vi "VectorField1008.vi"   [LabVIEW 2013]
uses:
  <vilib>/Heliosphere Research LLC/Advanced Plotting Toolkit/api_plotting/VectorFieldProperties.ctl
  <vilib>/Heliosphere Research LLC/Advanced Plotting Toolkit/typedefs/PlotColor.ctl
  <vilib>/Heliosphere Research LLC/Advanced Plotting Toolkit/properties/Colormap.ctl
  <vilib>/Heliosphere Research LLC/Advanced Plotting Toolkit/properties/Colormap_Map.ctl
  <vilib>/Heliosphere Research LLC/Advanced Plotting Toolkit/properties/Colormap_Scaling.ctl
  <vilib>/Heliosphere Research LLC/Advanced Plotting Toolkit/properties/Display.ctl
  <vilib>/Heliosphere Research LLC/Advanced Plotting Toolkit/Advanced Plotting Toolkit.lvlib
types:
  T1 = typedef "Advanced Plotting Toolkit.lvlib/Colormap_Map.ctl" = enum16{"Automatic", "Rainbow", "Hot and Cold", "White-Black", "White-Blue", "White-Green", "White-Red", "Fire", "Water", "Earth", "Air", "Pastel", "Banded", "Stepped"}
  T2 = typedef "Advanced Plotting Toolkit.lvlib/VectorFieldProperties.ctl" = cluster{"Color":T3, "Arrow Scale":dbl, "Colormap":T4, "Display":T6}
  T3 = typedef "Advanced Plotting Toolkit.lvlib/PlotColor.ctl" = u32
  T4 = typedef "Advanced Plotting Toolkit.lvlib/Colormap.ctl" = cluster{"Map":T1, "Value Min":dbl, "Value Max":dbl, "Scaling":T5, "Reverse":bool}
  T5 = typedef "Advanced Plotting Toolkit.lvlib/Colormap_Scaling.ctl" = enum16{"Default"}
  T6 = typedef "Advanced Plotting Toolkit.lvlib/Display.ctl" = cluster{"Alpha":dbl, "Z Order":dbl}
  T7 = typedef "Advanced Plotting Toolkit.lvlib/PlotID.ctl" = i32
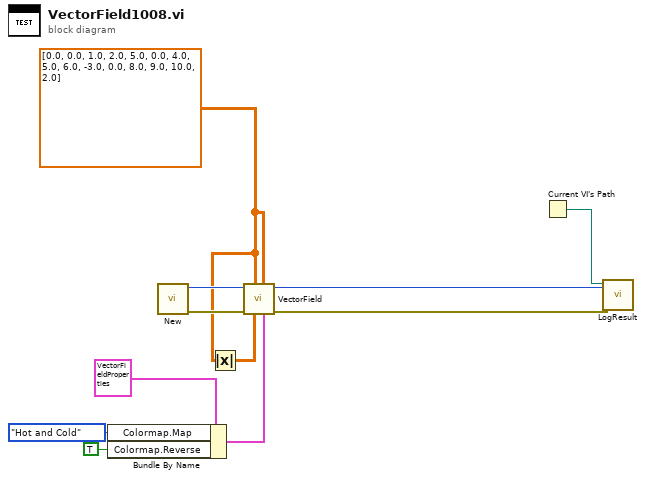
[diagram p0: block diagram]
diagram:
  w6 = dbl[][] [[0.0, 0.0, 1.0, 2.0, 5.0], [0.0, 4.0, 5.0, 6.0, -3.0], [0.0, 8.0, 9.0, 10.0, 2.0]] ("Data")
  n1 = Bundle By Name(cluster=T2 {"Color"=2147483647, "Arrow Scale"=nan, "Colormap"={"Map"=enum."Automatic", "Value Min"=nan, "Value Max"=nan, "Scaling"=enum."Default", "Reverse"=FALSE}, "Display"={"Alpha"=nan, "Z Order"=nan}} ("Vector Field Properties"), "Colormap.Map"=Colormap_Map."Hot and Cold", "Colormap.Reverse"=TRUE) -> (w3:T2)
  n2 = call <vilib>:"New.vi"() -> ("error out"=w9:errorcluster, "Plot ID"=w10:T7)  [unwired: 10 in]
  n3 = Absolute Value(x=w6) -> (abs(x)=w5:dbl[][])
  n4 = call <vilib>:"VectorField.vi"("Properties"=w3, "Y Vector Component"=w6, "Colormap Values"=w5, "X Vector Component"=w6, "error in (no error)"=w9, "Plot ID"=w10) -> ("error out"=w7:errorcluster, "Plot ID Out"=w8:T7)  [unwired: 4 in]
  n5 = Current VI's Path() -> (path=w11:path)
  n6 = call "LogResult.vi"("Test Result"=w7, "Test Artifact"=w8, "VI Path"=w11) -> ()  [unwired: 9 in]
